vi "send.vi"(8 "Error In":errorcluster, 9 "Severity Code (error)":T1=enum."error", 10 "Message Content":string, 11 "Message Tag":string) -> (0 "Error Out":errorcluster)   [LabVIEW 2013, in "CS++MessageLogger.lvlib"]
doc: "Send mesage to central message logger."
uses:
  CS++MessageLogger.lvlib
  Base/Severity.ctl
  <userlib>/syslog/_subVIs/TypeDefs/syslog_facility_codes.ctl
  Base/CS++Base.lvlib
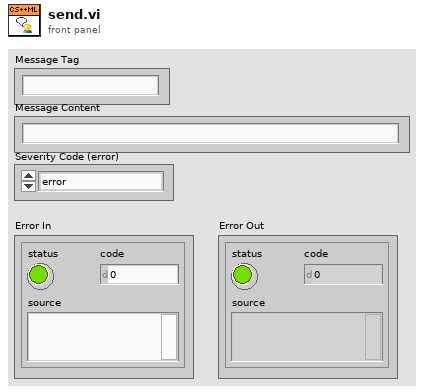
[diagram p1: front panel]
types:
  T1 = typedef "CS++Base.lvlib/Severity.ctl" = enum16{"emergency", "alert", "critical", "error", "warning", "notice", "info", "debug"}
  T2 = typedef "syslog_facility_codes.ctl" = enum16{"kernel", "user", "mail", "system daemons", "security/authorization", "syslogd", "line printer", "network news", "uucp", "clock daemon", "security/authorization (alternate)", "FTP daemon", "NTP subsystem", "log audit", "log alert", "clock daemon (alternate)", "local use 0", "local use 1", "local use 2", "local use 3", "local use 4", "local use 5", "local use 6", "local use 7"}
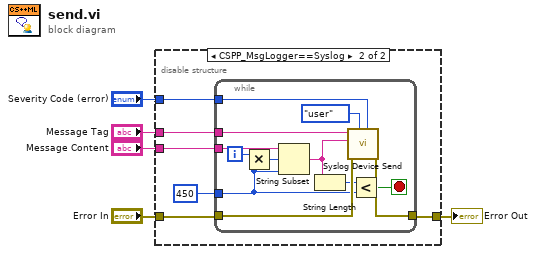
[diagram p0: block diagram]
diagram:
  n1 = disable-structure shown="CSPP_MsgLogger==Syslog" {
    disable-tunnel: "Message Tag" -> [_ w12]
    disable-tunnel: "Message Content" -> [_ w8]
    disable-tunnel: "Severity Code (error)" -> [_ w11]
    disable-tunnel: "Error In" -> [w6 w10]
    disable-tunnel: [w6 w9] -> w1
    frame condition #0 {
    }
    frame condition #1 (active) {
      n2 = while {
        tunnel: w12 -> [w24]
        tunnel: w11 -> [w22]
        tunnel: w10 -> [w21]
        tunnel: [w20] -> w9
        tunnel: w8 -> [w19]
        tunnel: 450 ("length (rest)") -> [w15]
        i -> [w18]
        stop <- w16 stop-if-true
        n3 = Multiply(x=w18, y=w15) -> (x*y=w17:i32)
        n4 = String Subset(string=w19, offset (0)=w17, length (rest)=w15) -> (substring=w13:string)
        n5 = String Length(string=w13) -> (length=w14:i32)
        n6 = call <userlib>:"Syslog Device Send.vi"("Severity Code (error)"=w22, "Facility Code (user)"=syslog_facility_codes."user", "error in (no error)"=w21, "Message Content"=w13, "Message Tag"=w24) -> ("error out"=w20:errorcluster)  [unwired: 5 in, 1 out]
        n7 = Less?(x=w14, y=w15) -> (x < y?=w16:bool)
      }
    }
  }
  "Error Out" <- w1
